vi "output.vi"(8 "error in":errorcluster, 10 "data table in":T1, 11 "Profibus Module runtime in":refnum<class "Profibus Module runtime.lvclass">) -> (0 "error out":errorcluster, 2 "data table out":T1, 3 "Profibus Module runtime out":refnum<class "Profibus Module runtime.lvclass">)   [LabVIEW 2013, in "Profibus Module runtime.lvclass"]
doc: "Provides an interface for writing data to a module at runtime. While this interface performs no operations, a child should provide an override which may write to any open sessions, references, or interfaces."
uses:
  Profibus Module runtime.lvclass
  <vilib>/NI/Tag Bus/table/data table.ctl
  Profibus Module runtime.lvclass/Profibus Module runtime.ctl
  dynamic profibus/dynamic profibus.lvlib
  <vilib>/NI/Tag Bus/table/data table.lvlib
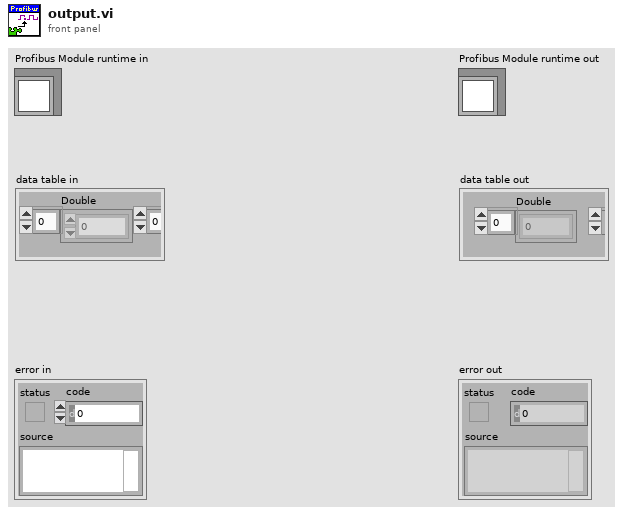
[diagram p1: front panel]
types:
  T1 = typedef "tag bus.lvlib/data table.lvlib/data table.ctl" = cluster{"Double":dbl[], "Single":sgl[], "I64":i64[], "I32":i32[], "I16":i16[], "I8":i8[], "U64":u64[], "U32":u32[], "U16":u16[], "U8":u8[], "Boolean":bool[], "String":string[], "Array of Double":cluster{"DBL Array":dbl[]}[], "Array of Single":cluster{"SGL Array":sgl[]}[], "Array of I64":cluster{"I64 Array":i64[]}[], "Array of I32":cluster{"I32 Array":i32[]}[], "Array of I16":cluster{"I16 Array":i16[]}[], "Array of I8":cluster{"I8 Array":i8[]}[], "Array of U64":cluster{"U64 Array":u64[]}[], "Array of U32":cluster{"U32 Array":u32[]}[], "Array of U16":cluster{"U16 Array":u16[]}[], "Array of U8":cluster{"U8 Array":u8[]}[], "Array of Boolean":cluster{"Boolean Array":bool[]}[], "Array of String":cluster{"String Array":string[]}[]}
  T2 = typedef "dynamic profibus.lvlib/fpga reference.ctl" = refnum<k20>
  T3 = typedef "dynamic profibus.lvlib/full command.ctl" = cluster{"action":T4, "device":u8, "index":u8, "data":u8}
  T4 = typedef "dynamic profibus.lvlib/profibus master action.ctl" = enum8{"initialize", "uninitialize", "stop", "get input", "get input size", "set output", "get output size", "get diagnostic", "transfer data", "transfer diagnostics"}
  T5 = typedef "Profibus Module runtime.lvclass/profibus slave configuration.ctl" = cluster{"slave index":i8, "data items":T6[], "data buffer":u8[], "big endian":bool, "data length":i32, "command list":T3[]}
  T6 = typedef "Profibus Module runtime.lvclass/profibus mapping configuration.ctl" = cluster{"data type":T7, " byte":i32, " bit":i32, "tag index":i32}
  T7 = typedef "tag bus.lvlib/tag descriptor.lvclass/Data Type.ctl" = enum16{"Double", "Single", "I64", "I32", "I16", "I8", "U64", "U32", "U16", "U8", "Boolean", "String", "Array of Double", "Array of Single", "Array of I64", "Array of I32", "Array of I16", "Array of I8", "Array of U64", "Array of U32", "Array of U16", "Array of U8", "Array of Boolean", "Array of String"}
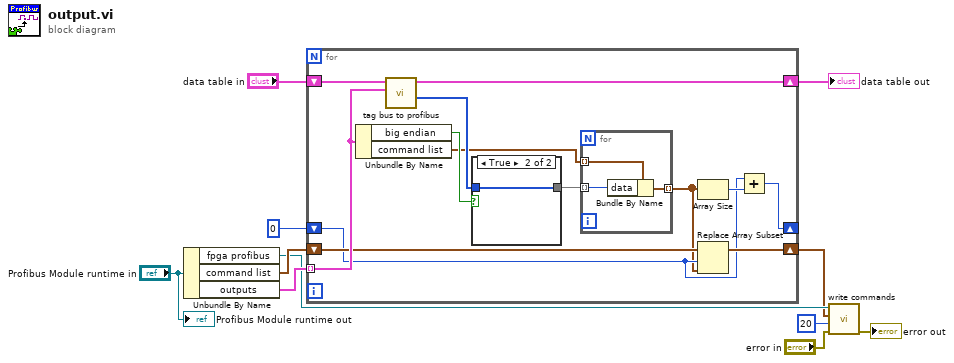
[diagram p0: block diagram]
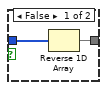
[diagram p2: hidden frame]
diagram:
  n1 = Unbundle By Name("Profibus Module runtime in") -> ("fpga profibus"=w2:T2, "command list"=w7:T3[], "outputs"=w9:T5[])
  n2 = for {
    shift-right: [w23] -> w10
    shift-left: "data table in" -> [w24]
    tunnel: w9 -> [w22] mode=indexing
    shift-right: [w14] -> w1
    shift-left: w7 -> [w15]
    shift-right: [w16] -> _
    shift-left: 0 -> [w13]
    n3 = Unbundle By Name(w22) -> ("big endian"=w21:bool, "command list"=w18:T3[])
    n4 = call "tag bus to profibus.vi"("slave configuration"=w22, "data table in in"=w24) -> ("Data"=w20:u8[], "data table out"=w23:T1)  [unwired: 7 in, 1 out]
    n5 = case shown="True" w21 {
      tunnel: [w28 w30] -> w19
      tunnel: w20 -> [w29 w30]
      frame False {
        n6 = Reverse 1D Array(array=w29) -> (reversed array=w28:u8[])
      }
      frame True {
      }
    }
    n7 = for {
      tunnel: w19 -> [w26] mode=indexing
      tunnel: w18 -> [w27] mode=indexing
      tunnel: [w25] -> w12 mode=indexing
      n8 = Bundle By Name(cluster=w27, "data"=w26) -> (w25:T3)
    }
    n9 = Array Size(array=w12) -> (size(s)=w17:i32)
    n10 = Replace Array Subset(array=w15, new element=w12, index=w13) -> (w14:T3[])
    n11 = Add(x=w13, y=w17) -> (x+y=w16:i32)
  }
  "data table out" <- w10
  n12 = call "write commands.vi"("error in"="error in", "Timeout (ms)"=20, "commands"=w1, "profibus reference"=w2) -> ("error out"=→"error out":errorcluster)  [unwired: 6 in, 1 out]
  "Profibus Module runtime out" <- "Profibus Module runtime in"
